vi "Persist Config.vi"(7 "Overlay Filters (None)":refnum<class "Overlay Filter.lvclass">[](array[class]), 8 "error in (no error)":errorcluster, 10 "Config":refnum<class "Config Manager.lvclass">, 11 "Config Storage in":refnum<class "Config Storage.lvclass">) -> (0 "error out":errorcluster, 3 "Config Storage out":refnum<class "Config Storage.lvclass">)   [LabVIEW 2020, in "CDM-Config.lvlib" / "Config Storage.lvclass"]
uses:
  Config Storage.lvclass
  Config Manager/Config Manager.lvclass
  Overlay Filter/Overlay Filter.lvclass
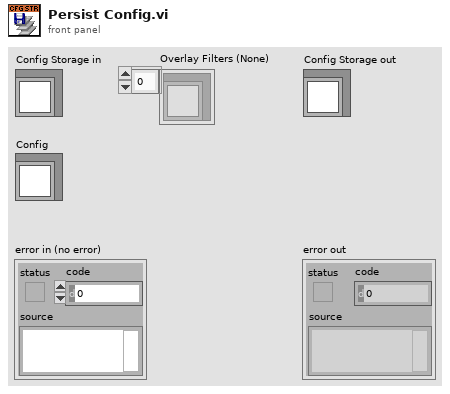
[diagram p1: front panel]
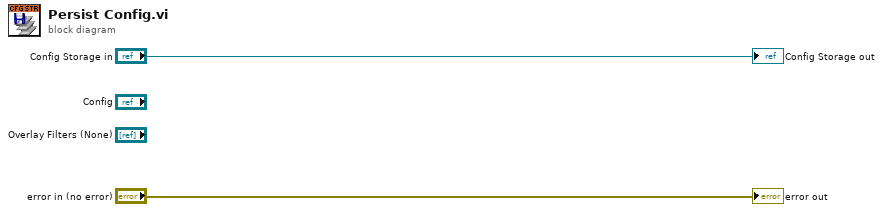
[diagram p0: block diagram]
diagram:
  "error out" <- "error in (no error)"
  "Config Storage out" <- "Config Storage in"
